vi "JSON to Cluster Preparation.vi"(8 "error in (no error)":errorcluster, 11 "Cluster":variant) -> (0 "error out":errorcluster, 1 "Element Info":T3(array[cluster]), 2 "Elements":variant[](array[variant]), 3 "ELement Names (as JSON)":string[](array[string]))   [LabVIEW 2024, in "JSONtext.lvlib"]
uses:
  JSONtext.lvlib
  Data Type.ctl
  Tag Type.ctl
  quote and escape json string 2.vi
  NI_Data Type.lvlib
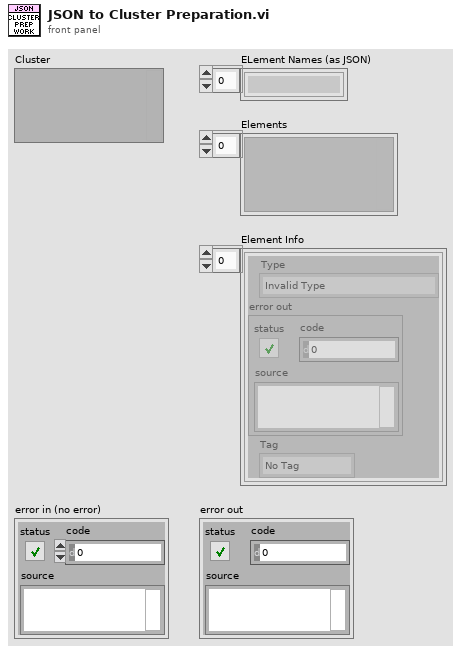
[diagram p1: front panel]
types:
  T1 = typedef "NI_Data Type.lvlib/Data Type.ctl" = enum8{"Invalid Type", "Void", "I8", "I16", "I32", "I64", "U8", "U16", "U32", "U64", "Single Float", "Double Float", "Extended Float", "Single Complex", "Double Complex", "Extended Complex", "Enum U8", "Enum U16", "Enum U32", "Enum U64", "Single Float With Unit", "Double Float With Unit", "Extended Float With Unit", "Single Complex with Unit", "Double Complex with Unit", "Extended Complex with Unit", "Boolean", "String", "Path", "Picture", "Tag", "Array", "Cluster", "Variant", "LV Variant", "Waveform", "Timestamp", "Digital Waveform", "Digital Data", "ExpressData", "Refnum", "External Data", "VI", "Poly VI", "LabVIEW Class Instance", "Fixed Point", "Set Collection", "Map Collection"}
  T2 = typedef "JSONtext.lvlib/Tag Type.ctl" = enum16{"No Tag", "<JSON>", "<JOBJ>", "<UTF8>"}
  T3 = cluster{"Type":T1, "error out":errorcluster, "Tag":T2}[]
  T4 = cluster{"type":T1, "error out":errorcluster, "Tag":T2}
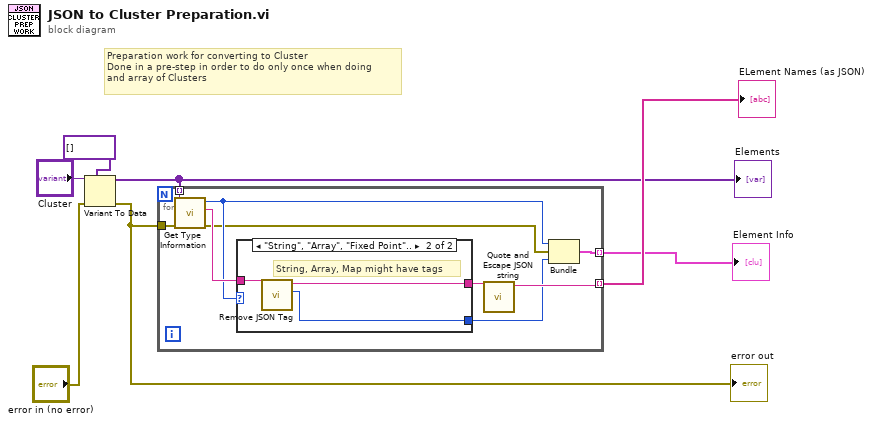
[diagram p0: block diagram]
diagram:
  # "Preparation work for converting to Cluster\nDone in a pre-step in order to do only once when doing\nand array of Clusters"
  n1 = Variant To Data(error in="error in (no error)", type=variant[] [], Variant="Cluster") -> (data=w5:variant[], error out=w4:errorcluster)
  "Elements" <- w5
  "error out" <- w4
  n2 = for {
    tunnel: w5 -> [w16] mode=indexing
    tunnel: w4 -> [w15]
    tunnel: [w8] -> w6 mode=indexing
    tunnel: [w13] -> w7 mode=indexing
    n3 = call "Get Type Information.vi"("error in (no error)"=w15, "variant"=w16) -> ("error out"=w9:errorcluster, "name"=w14:string, "type"=w11:T1)  [unwired: 5 in, 2 out]
    n4 = case shown="\"String\", \"Array\", \"Fixed Point\".." w11 {
      tunnel: w14 -> [w17 w20]
      tunnel: [_ w19] -> w10
      tunnel: [w17 w18] -> w12
      frame Default {
      }
      frame "String", "Array", "Fixed Point".. {
        # "String, Array, Map might have tags"
        n5 = call "Remove JSON Tag.vi"("Name"=w20) -> ("Tag"=w19:T2, "Name (tag stripped)"=w18:string)  [unwired: 9 in]
      }
    }
    n6 = call "Quote and Escape JSON string.vi"("Plain Text"=w12) -> ("<JSON>"=w13:string)  [unwired: 10 in]
    n7 = Bundle("type"=w11, "error out"=w9, "Tag"=w10) -> (w8:T4)  [unwired: 1 in]
  }
  "ELement Names (as JSON)" <- w7
  "Element Info" <- w6
